vi "WhileLoop-Ver2.vi"() -> ()   [LabVIEW 2018]
panel:
  out "Maximum Value of Count":dbl
  out "Value from Dial":dbl
  out "Count from Loop":dbl
  in  "Maximum Number":dbl(knob) scale=0.0..20.0
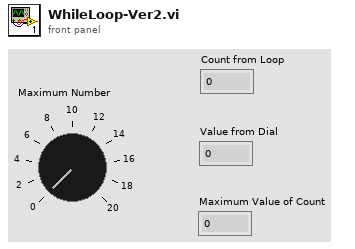
[diagram p1: front panel]
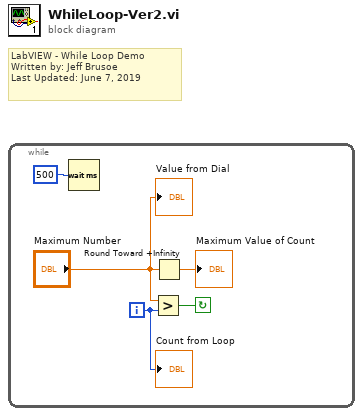
[diagram p0: block diagram]
diagram:
  # "LabVIEW - While Loop Demo\nWritten by: Jeff Brusoe\nLast Updated: June 7, 2019"
  n1 = while {
    i -> [w5]
    stop <- w3 continue-if-true
    n2 = Wait (ms)(milliseconds to wait=500) -> ()  [unwired: 1 out]
    n3 = Greater?(x="Maximum Number", y=w5) -> (0:w3:bool)
    n4 = Round Toward +Infinity(x="Maximum Number") -> (ceil(x): smallest int >= x=→"Maximum Value of Count":dbl)
    "Count from Loop" <- w5
    "Value from Dial" <- "Maximum Number"
  }
